vi "Get Exported Tag Path.vi"(11 "channel name":string) -> (3 "tag path":string)   [LabVIEW 2020, in "FlexLoggerTagHelpers.lvlib"]
uses:
  FlexLoggerTagHelpers.lvlib
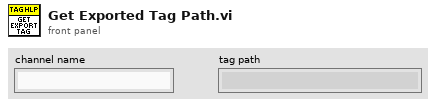
[diagram p1: front panel]
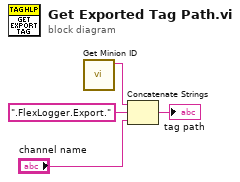
[diagram p0: block diagram]
diagram:
  n1 = call <vilib>:"Get Minion ID.vi"() -> ("minion id"=w3:string)  [unwired: 11 in]
  n2 = Concatenate Strings(w3, ".FlexLogger.Export." ("string"), "channel name") -> (→"tag path":string)
